vi "Force.vi"(8 "error in (no error)":errorcluster, 9 "Device and Axis":string, 10 "Output Force (0)":i32 min=-700 max=700, 11 "VISA resource name":refnum<visa-resource-name>) -> (0 "error out":errorcluster, 3 "VISA resource name out":refnum<visa-resource-name>)   [LabVIEW 2018, in "Zaber A Series.lvlib"]
doc: "Set the continuous force output on Zaber devices that support force output mode, such as the X-DMQ-DE voice coil. \n\nThe Output Force value is in a unitless device-specific resolution; consult your device manual for the conversion from standard force units. \n\nContinuous force output can be combined with sinusoidal force produced by the Sinusoidal Force VI. Input a force of zero to turn off continuous force output without interrupting the sinusoid, or use the Force Off VI to disable both at once.\n\nThis VI requires that the VISA serial port input has already been configured and opened."
uses:
  Zaber A Series.lvlib
  Private/All Commands.ctl
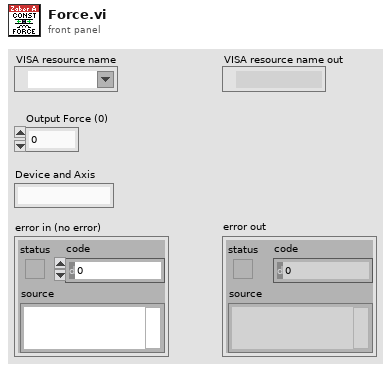
[diagram p1: front panel]
types:
  T1 = typedef "Zaber A Series.lvlib/All Commands.ctl" = string
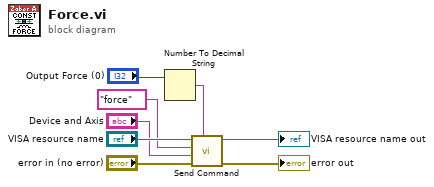
[diagram p0: block diagram]
diagram:
  n1 = Number To Decimal String(number="Output Force (0)") -> (decimal integer string=w3:string)  [unwired: 1 in]
  n2 = call "Send Command.vi"("Data"=w3, "error in (no error)"="error in (no error)", "Device and Axis"="Device and Axis", "Command"=T1 "force" ("Complete Command List"), "VISA resource name"="VISA resource name") -> ("error out"=→"error out":errorcluster, "VISA resource name out"=→"VISA resource name out":refnum<visa-resource-name>)  [unwired: 1 in, 4 out]
